vi "ToggleMainCameraView.vi"(11 "Enable? (T)":bool=TRUE) -> ()   [LabVIEW 2011]
uses:
  GlobalVariables.vi
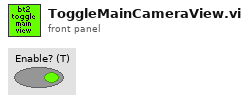
[diagram p1: front panel]
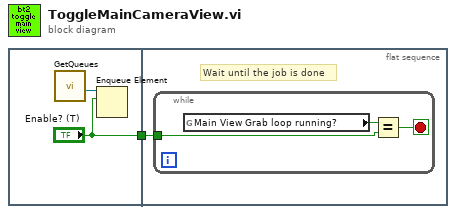
[diagram p0: block diagram]
diagram:
  n1 = flat-sequence {
    tunnel: ["Enable? (T)"] -> w1
    tunnel: w1 -> [w4]
    frame #0 {
      n2 = call "GetQueues.vi"() -> ("User Interface Camera Control"=w3:refnum<queue>)  [unwired: 10 in, 1 out]
      n3 = Enqueue Element(queue=w3, element="Enable? (T)") -> ()  [unwired: 2 in, 3 out]
    }
    frame #1 {
      # "Wait until the job is done"
      n4 = while {
        tunnel: w4 -> [w6]
        stop <- w5 stop-if-true
        n5 = global read "GlobalVariables.vi" "Main View Grab loop running?"() -> (w7:bool)
        n6 = Equal?(x=w7, y=w6) -> (x = y?=w5:bool)
      }
    }
  }
